vi "test_generator.vi"() -> ()   [LabVIEW 2014]
panel:
  in  "pause":bool
  in  "triangle_control":T1 {"end_source / V" format="%#_13g"; "lower_volt_limit / V" format="%#_13g"; "upper_volt_limit / V" format="%#_13g"; "step_voltage / V" format="%#_13g"; "init_source / V" format="%#_13g"}
  out "Waveform Chart":dbl(graph)
  in  "stop":bool
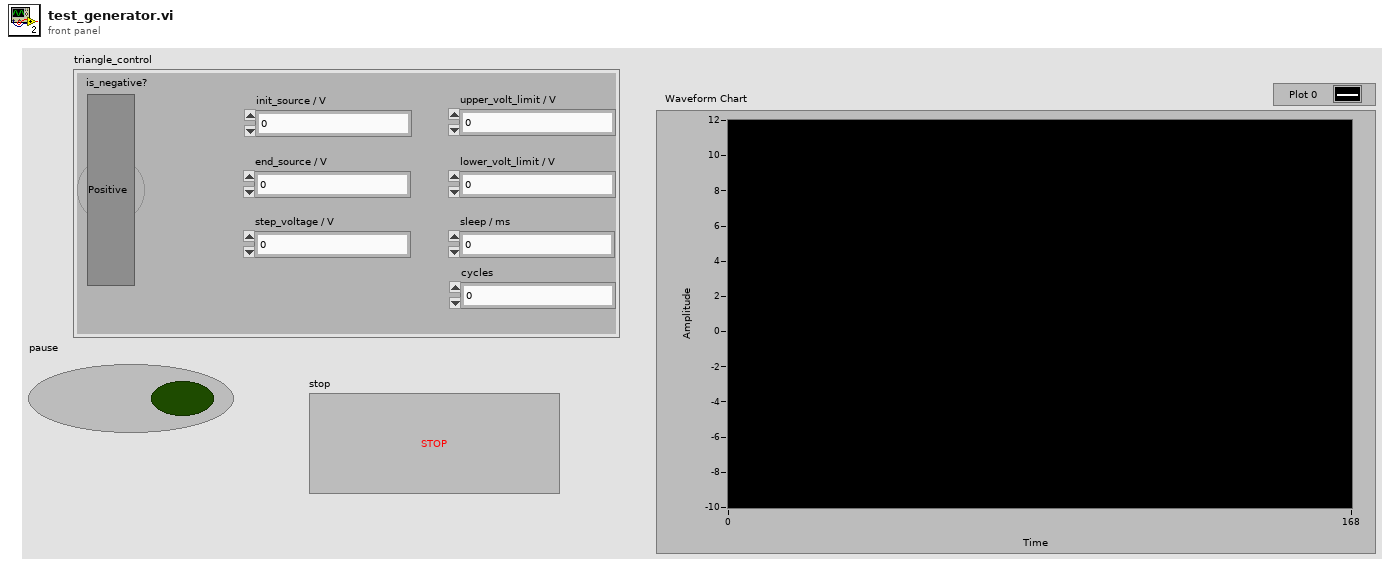
[diagram p1: front panel]
types:
  T1 = cluster{"init_source / V":dbl, "step_voltage / V":dbl, "upper_volt_limit / V":dbl, "lower_volt_limit / V":dbl, "sleep / ms":u32, "is_negative?":bool, "cycles":u32, "end_source / V":dbl}
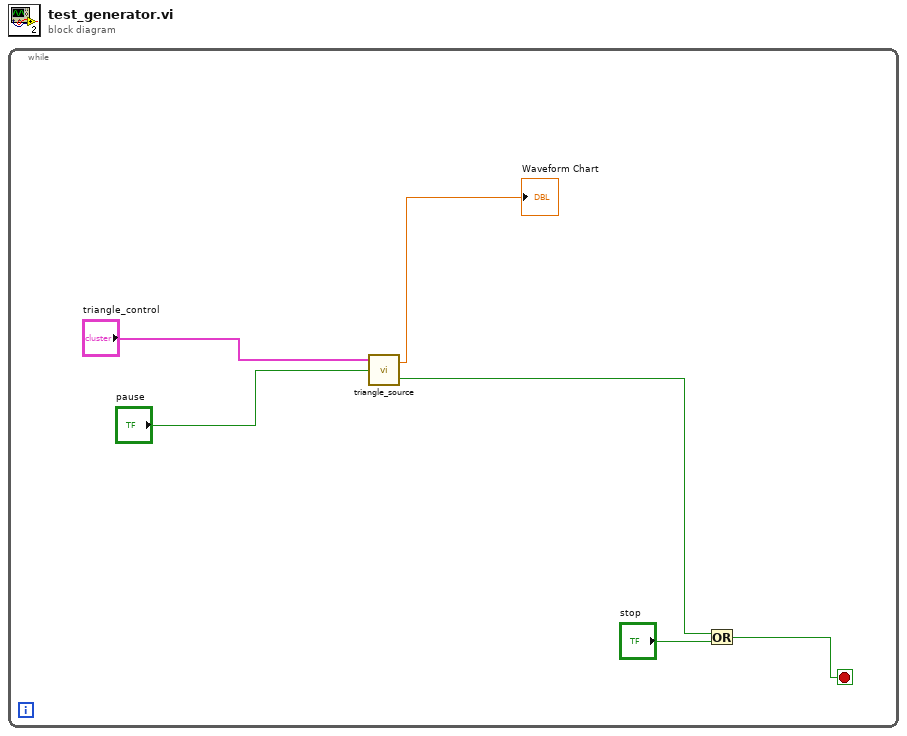
[diagram p0: block diagram]
diagram:
  n1 = while {
    stop <- w5 stop-if-true
    n2 = call "triangle_source.vi"("pause"="pause", "triangle_control"="triangle_control") -> ("terminate?"=w2:bool, "output_signal / V"=→"Waveform Chart":dbl)  [unwired: 1 in]
    n3 = Or(x=w2, y="stop") -> (x .or. y?=w5:bool)
  }
